vi "Get Session Info - NSess .vi"(8 "error in":errorcluster, 11 "session reservation in":refnum<class "Session Reservation.lvclass">) -> (0 "error out":errorcluster, 2 "sessions info":T1[](array[typedef]), 3 "session reservation out":refnum<class "Session Reservation.lvclass">)   [LabVIEW 2020, in "MeasurementLink Session Management V1.lvlib" / "Session Reservation.lvclass"]
doc: "Gets the session information for the session reservation."
uses:
  Session Reservation.lvclass
  MeasurementLink Session Management Client/RPC Messages/ni_measurementlink_sessionmanagement_v1_SessionInformation.ctl
  MeasurementLink Session Management Client/RPC Messages/nidevice_grpc_Session.ctl
  MeasurementLink Session Management Client/RPC Messages/ni_measurementlink_sessionmanagement_v1_ChannelMapping.ctl
  Session Reservation.lvclass/Session Reservation.ctl
  MeasurementLink Measurement Server/Helpers/Error Strings Global Internal.vi
  <vilib>/Utility/error.llb/Error Cluster From Error Code.vi
  MeasurementLink Session Management Client/MeasurementLink Session Management Client.lvlib
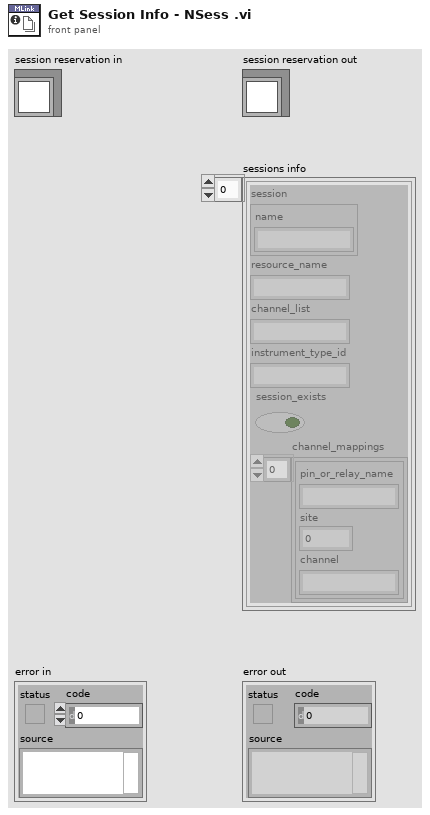
[diagram p1: front panel]
types:
  T1 = typedef "MeasurementLink Session Management Client.lvlib/ni_measurementlink_sessionmanagement_v1_SessionInformation.ctl" = cluster{"session":T2, "resource_name":string, "channel_list":string, "instrument_type_id":string, "session_exists":bool, "channel_mappings":T3[]}
  T2 = typedef "MeasurementLink Session Management Client.lvlib/nidevice_grpc_Session.ctl" = cluster{"name":string}
  T3 = typedef "MeasurementLink Session Management Client.lvlib/ni_measurementlink_sessionmanagement_v1_ChannelMapping.ctl" = cluster{"pin_or_relay_name":string, "site":i32, "channel":string}
  T4 = typedef "MeasurementLink Session Management V1.lvlib/Session Reservation.lvclass/Data.ctl" = cluster{"session and driver infos":T5[], "pin or relay names":string[], "connection map":refnum<class "Connection Map.lvclass">, "pin map context":T7, "reservation observer":refnum<class "IReservationObserver.lvclass">, "dvr valid":bool}
  T5 = typedef "MeasurementLink Session Management V1.lvlib/Session Reservation.lvclass/Session and Driver Info.ctl" = cluster{"session info":T1, "session":variant, "session factory":refnum<class "ISession Factory.lvclass">, "initialize and close session behavior":T6}
  T6 = typedef "MeasurementLink Instrument.lvlib/ISession Factory.lvclass/Initialize and Close Session Behavior.ctl" = enum16{"Initialize and Close", "Attach and Detach", "Initialize and Detach", "Attach and Close"}
  T7 = typedef "MeasurementLink Session Management Client.lvlib/ni_measurementlink_PinMapContext.ctl" = cluster{"pin_map_id":string, "sites":i32[]}
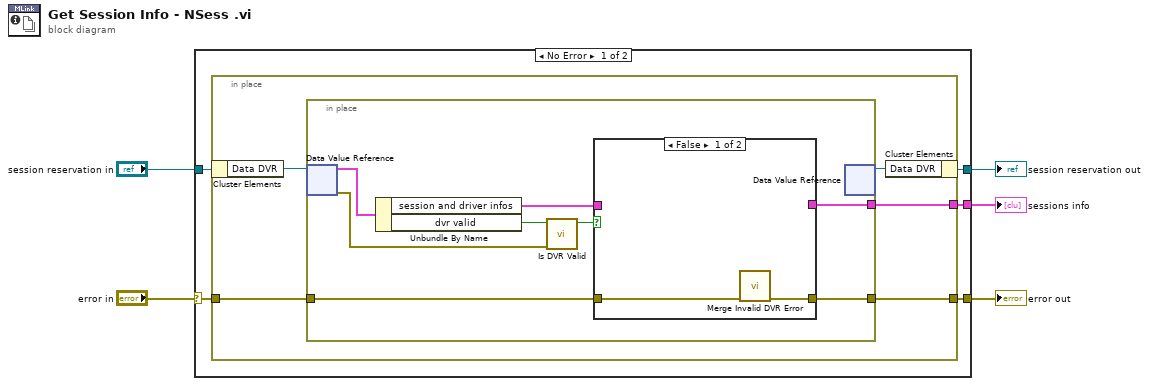
[diagram p0: block diagram]
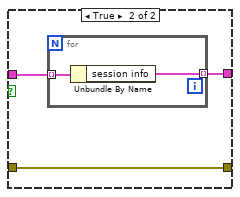
[diagram p2: hidden frame]
diagram:
  n1 = case shown="No Error" "error in" {
    selector: "error in" -> [w6 w32]
    tunnel: "session reservation in" -> [w10 w31]
    tunnel: [w9 w31] -> w4
    tunnel: [w8 _] -> w3
    tunnel: [w7 w32] -> w2
    frame No Error {
      n2 = in-place {
        in-place-border: [w15] -> w7
        in-place-border: [w12] -> w8
        in-place-border: w6 -> [w11]
        n3 = in-place-cluster #1(w10) -> ("Data DVR"=w14:refnum<data-value>)
        n4 = in-place {
          in-place-border: w11 -> [w23]
          in-place-border: [w22] -> w15
          in-place-border: [w19] -> w12
          n5 = in-place-dvr #2(w14) -> (w20:T4, w16:errorcluster)
          n6 = Unbundle By Name(w20) -> ("session and driver infos"=w21:T5[], "dvr valid"=w18:bool)
          n7 = call "Is DVR Valid.vi"("dvr error in"=w16, "dvr valid"=w18) -> ("dvr valid"=w17:bool)  [unwired: 9 in]
          n8 = case shown="False" w17 {
            tunnel: w23 -> [w25 w28]
            tunnel: [w24 w28] -> w22
            tunnel: w21 -> [_ w27]
            tunnel: [_ w26] -> w19
            frame False {
              n9 = call "Merge Invalid DVR Error.vi"("error in (no error)"=w25) -> ("error out"=w24:errorcluster)  [unwired: 10 in]
            }
            frame True {
              n10 = for {
                tunnel: w27 -> [w30] mode=indexing
                tunnel: [w29] -> w26 mode=indexing
                n11 = Unbundle By Name(w30) -> ("session info"=w29:T1)
              }
            }
          }
          n12 = in-place-dvr #2() -> (w13:refnum<data-value>)  [unwired: 1 in, 1 out]
        }
        n13 = in-place-cluster #1("Data DVR"=w13) -> (w9:refnum<class "Session Reservation.lvclass">)
      }
    }
    frame Error {
    }
  }
  "error out" <- w2
  "session reservation out" <- w4
  "sessions info" <- w3
